vi "XY to BoundingBox for Drawing Spots.vi"(2 "Radius":dbl=3.0 format="%#_13g", 3 "Central Coords":cluster{dbl, dbl}) -> (0 "Bounding Box":cluster{dbl, dbl, dbl, dbl})   [LabVIEW 2020]
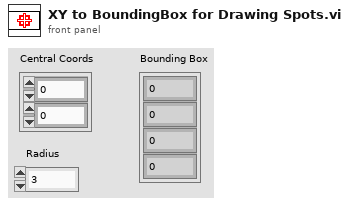
[diagram p1: front panel]
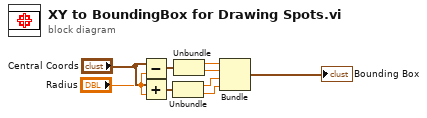
[diagram p0: block diagram]
diagram:
  n1 = Subtract(x="Central Coords", y="Radius") -> (x-y=w2:cluster{dbl, dbl})
  n2 = Add(x="Central Coords", y="Radius") -> (x+y=w3:cluster{dbl, dbl})
  n3 = Unbundle(w3) -> (w6:dbl, w7:dbl)
  n4 = Unbundle(w2) -> (w4:dbl, w5:dbl)
  n5 = Bundle(w4, w5, w6, w7) -> (→"Bounding Box":cluster{dbl, dbl, dbl, dbl})  [unwired: 1 in]
